vi "Set polarity.vi"(8 "error in":errorcluster, 10 "Polarity":i16(ring)=1 items=["POSITIVE"=1, "NEGATIVE"=-1], 11 "VISA resource name":refnum<visa-resource-name>) -> (0 "error out":errorcluster, 3 "VISA resource name out":refnum<visa-resource-name>)   [LabVIEW 2012, in "Datron D4xxx.lvlib"]
doc: "This VI allows you to change output polarity without value modification in DC modes."
uses:
  Datron D4xxx.lvlib
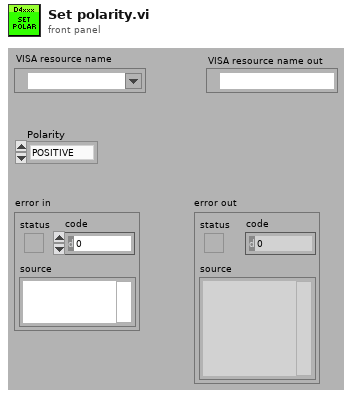
[diagram p1: front panel]
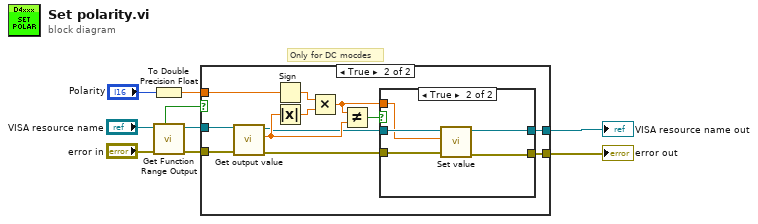
[diagram p0: block diagram]
diagram:
  # "Only for DC mocdes"
  n1 = To Double Precision Float(number="Polarity") -> (double precision float=w3:dbl)
  n2 = call "Get Function Range Output.vi"("error in (no error)"="error in", "VISA resource name"="VISA resource name") -> ("error out"=w4:errorcluster, "VISA resource name out"=w5:refnum<visa-resource-name>, "DC"=w6:bool)  [unwired: 2 in, 5 out]
  n3 = case shown="True" w6 {
    tunnel: w5 -> [w11 w23]
    tunnel: w4 -> [w10 w22]
    tunnel: w3 -> [_ w21]
    tunnel: [w10 w14] -> w2
    tunnel: [w11 w13] -> w1
    frame False {
    }
    frame True {
      n4 = call "Get output value.vi"("error in (no error)"=w22, "VISA resource name"=w23) -> ("error out"=w17:errorcluster, "Value"=w18:dbl, "VISA resource name out"=w16:refnum<visa-resource-name>)  [unwired: 7 in]
      n5 = Sign(1:w21) -> (0:w19:dbl)
      n6 = Absolute Value(x=w18) -> (abs(x)=w20:dbl)
      n7 = Multiply(x=w19, y=w20) -> (x*y=w12:dbl)
      n8 = Not Equal?(x=w12, y=w18) -> (x != y?=w15:bool)
      n9 = case shown="True" w15 {
        tunnel: w17 -> [w24 w30]
        tunnel: w16 -> [w25 w29]
        tunnel: [w24 w27] -> w14
        tunnel: [w25 w26] -> w13
        tunnel: w12 -> [_ w28]
        frame False {
        }
        frame True {
          n10 = call "Set value.vi"("error in"=w30, "Value"=w28, "VISA resource name"=w29) -> ("error out"=w27:errorcluster, "VISA resource name out"=w26:refnum<visa-resource-name>)  [unwired: 6 in, 1 out]
        }
      }
    }
  }
  "VISA resource name out" <- w1
  "error out" <- w2
